vi "Get Implementors.vi"(8 "error in (no error)":errorcluster, 11 "Dynamic Dispatch VI Type in":refnum<class "Dynamic Dispatch VI Type.lvclass">) -> (0 "error out":errorcluster, 2 "All Classes":refnum<vi>[](array[refnum]), 3 "Dynamic Dispatch VI Type out":refnum<class "Dynamic Dispatch VI Type.lvclass">)   [LabVIEW 2020, in "Peek Window.lvlib" / "Dynamic Dispatch VI Type.lvclass"]
uses:
  Dynamic Dispatch VI Type.lvclass
  D:/Code/VI-Peek/source/Peek Window/VI Types/Standard VI Type/Standard VI Type.lvclass
  Implementor Tree Item Info.ctl
  Implementation VI Type/Implementation VI Type.lvclass
  Standard VI Type/Standard VI Type.lvclass/Standard VI Type.ctl
  Dynamic Dispatch VI Type.lvclass/Dynamic Dispatch VI Type.ctl
  Standard VI Type/Write Full Qualified Name.vi
  Standard VI Type/Write App Refnum.vi
  Standard VI Type/Write VI Refnum.vi
  Standard VI Type/Write Openable.vi
  Standard VI Type/Write Selectable.vi
  Standard VI Type/Read App Refnum.vi
  Standard VI Type/Read Full Qualified Name.vi
  <vilib>/regexp/Match Regular Expression.xnode
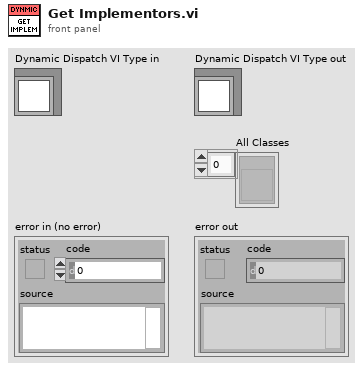
[diagram p1: front panel]
types:
  T1 = map{string, refnum<class "Implementation VI Type.lvclass">}
  T2 = typedef "Peek Window.lvlib/Dynamic Dispatch VI Type.lvclass/Implementor Tree Item Info.ctl" = cluster{"ClassRef":refnum<vi>, "Implementor?":bool, "Parent ItemID":string, "Full Qualified Name":string}
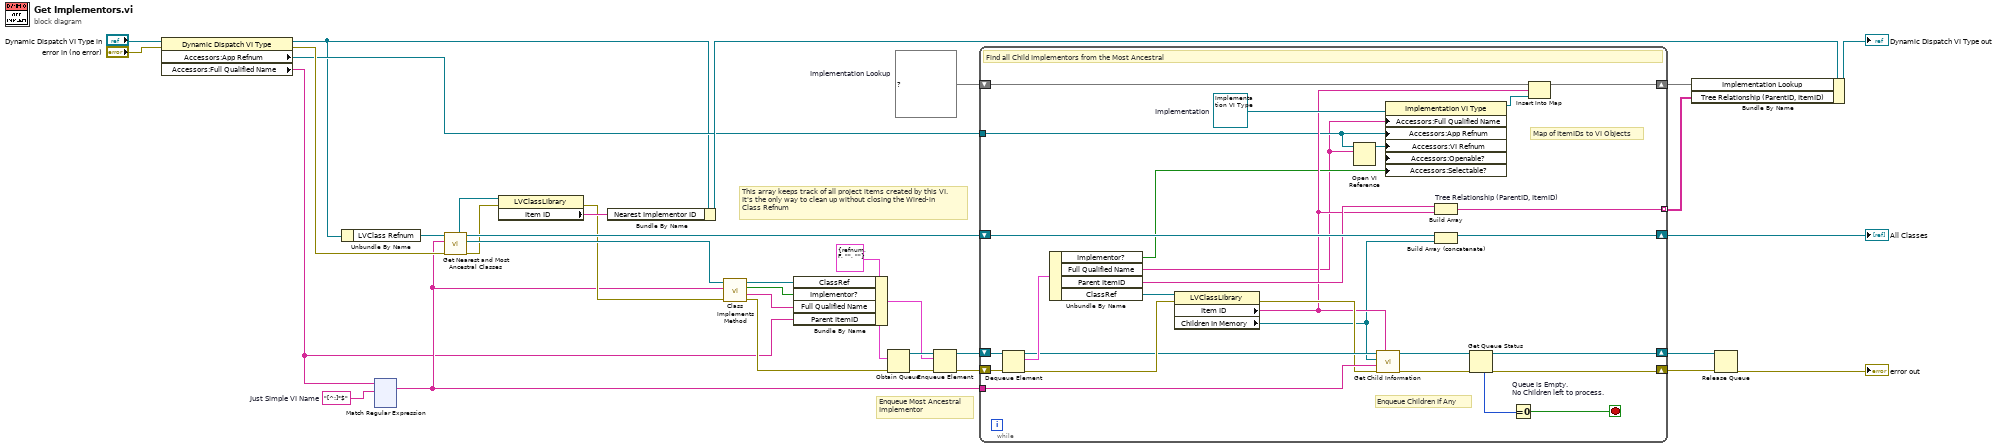
[diagram p0: block diagram]
diagram:
  w1 = "[^:]*$"  # Just Simple VI Name
  w25 = T1 {}  # Implementation Lookup
  w29 = T2 {"ClassRef"=refnum, "Implementor?"=FALSE, "Parent ItemID"="", "Full Qualified Name"=""} ("Cluster")
  # "Enqueue Most Ancestral\nImplementor"
  # "This array keeps track of all project items created by this VI.\nIt's the only way to clean up without closing the Wired-in \nClass Refnum"
  n1 = property class="Dynamic Dispatch VI Type"(reference="Dynamic Dispatch VI Type in", error in="error in (no error)") -> (reference out=w4:refnum<class "Dynamic Dispatch VI Type.lvclass">, error out=w11:errorcluster, "Accessors:App Refnum"=w10:refnum<vi>, "Accessors:Full Qualified Name"=w2:string)
  n2 = Unbundle By Name(w4) -> ("LVClass Refnum"=w5:refnum<vi>)
  n3 = xnode "Match Regular Expression"("input string"=w2, "regular expression"=w1) -> ("whole match"=w3:string)  [unwired: 4 in, 4 out]
  n4 = call "Get Nearest and Most Ancestral Classes.vi"("error in (no error)"=w11, "Simple Method Name"=w3, "Input Class Ref"=w5) -> ("error out"=w8:errorcluster, "Most Ancestral Class Ref"=w26:refnum<vi>, "All Class Refnums"=w14:refnum<vi>[], "Nearest Implementor Class Ref"=w13:refnum<vi>)  [unwired: 5 in]
  n5 = property class="LVClassLibrary"(reference=w13, error in=w8) -> (error out=w7:errorcluster, "Item ID"=w16:string)  [unwired: 1 out]
  n6 = Bundle By Name(cluster=w4, "Nearest Implementor ID"=w16) -> (w17:refnum<class "Dynamic Dispatch VI Type.lvclass">)
  n7 = call "Class Implements Method.vi"("error in (no error)"=w7, "Method Name"=w3, "Class Refnum"=w26) -> ("error out"=w23:errorcluster, "VI Qualified Name"=w22:string, "Implements method?"=w21:bool, "Class Refnum out"=w20:refnum<vi>)  [unwired: 5 in]
  n8 = Bundle By Name(cluster=w29, "ClassRef"=w20, "Implementor?"=w21, "Full Qualified Name"=w22, "Parent ItemID"=w2) -> (w32:T2)
  n9 = Obtain Queue(element data type=w29, error in (no error)=w23) -> (queue out=w34:refnum<queue>, error out=w33:errorcluster)  [unwired: 3 in, 1 out]
  n10 = Enqueue Element(queue=w34, element=w32, error in (no error)=w33) -> (queue out=w31:refnum<queue>, error out=w30:errorcluster)  [unwired: 1 in, 1 out]
  n11 = while {
    shift-right: [w43] -> w24
    shift-left: w30 -> [w61]
    tunnel: w3 -> [w53]
    shift-right: [w46] -> w27
    shift-left: w14 -> [w54]
    shift-right: [w48] -> w18
    shift-left: w25 -> [w49]
    shift-right: [w52] -> w28
    shift-left: w31 -> [w62]
    tunnel: [w40] -> w15 mode=indexing
    tunnel: w10 -> [w38]
    stop <- w60 stop-if-true
    w45 = refnum<class "Implementation VI Type.lvclass"> refnum  # Implementation
    # "Enqueue Children If Any"
    # "Map of ItemIDs to VI Objects"
    # "Find all Child Implementors from the Most Ancestral"
    n12 = Dequeue Element(queue=w62, error in (no error)=w61) -> (queue out=w56:refnum<queue>, element=w58:T2, error out=w57:errorcluster)  [unwired: 1 in, 1 out]
    n13 = Unbundle By Name(w58) -> ("Implementor?"=w39:bool, "Full Qualified Name"=w36:string, "Parent ItemID"=w42:string, "ClassRef"=w47:refnum<vi>)
    n14 = property class="LVClassLibrary"(reference=w47, error in=w57) -> (error out=w51:errorcluster, "Item ID"=w41:string, "Children In Memory"=w35:refnum<vi>[])  [unwired: 1 out]
    n15 = Open VI Reference(application reference (local)=w38, vi path=w36) -> (vi reference=w37:refnum<vi>)  [unwired: 4 in, 1 out]
    n16 = call "Get Child Information.vi"("ParentID"=w41, "error in (no error)"=w51, "Plain Method Name in"=w53, "Children in Memory"=w35, "Queue in"=w56) -> ("error out"=w50:errorcluster, "Queue out"=w55:refnum<queue>)  [unwired: 5 in]
    n17 = property class="Implementation VI Type"(reference=w45, "Accessors:Full Qualified Name"=w36, "Accessors:App Refnum"=w38, "Accessors:VI Refnum"=w37, "Accessors:Openable?"=w39, "Accessors:Selectable?"=w39) -> (reference out=w44:refnum<class "Implementation VI Type.lvclass">)  [unwired: 1 in, 1 out]
    n18 = Build Array "Tree Relationship (ParentID, ItemID)"(w42, w41) -> (w40:string[])
    n19 = Build Array (concatenate)(w54, w35) -> (w46:refnum<vi>[])
    n20 = Get Queue Status(queue=w55, error in (no error)=w50) -> (queue out=w52:refnum<queue>, error out=w43:errorcluster, # elements in queue=w59:i32)  [unwired: 1 in, 5 out]
    n21 = Equal To 0? "Queue is Empty.  \nNo Children left to process."(x=w59) -> (x = 0?=w60:bool)
    n22 = Insert Into Map(map in=w49, key=w41, value=w44) -> (map out=w48:T1)  [unwired: 2 out]
  }
  "All Classes" <- w27
  n23 = Bundle By Name(cluster=w17, "Implementation Lookup"=w18, "Tree Relationship (ParentID, ItemID)"=w15) -> (→"Dynamic Dispatch VI Type out":refnum<class "Dynamic Dispatch VI Type.lvclass">)
  n24 = Release Queue(queue=w28, error in (no error)=w24) -> (error out=→"error out":errorcluster)  [unwired: 1 in, 2 out]
